vi "sync.create.vi"(8 "error in (no error)":errorcluster) -> (0 "error out":errorcluster, 3 "synchronization":refnum<class "synchronization.lvclass">)   [LabVIEW 2020, in "synchronization.lvclass"]
uses:
  synchronization.lvclass
  synchronization.lvclass/synchronization.ctl
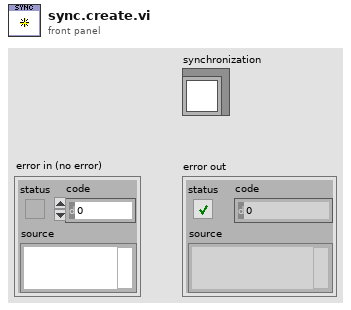
[diagram p1: front panel]
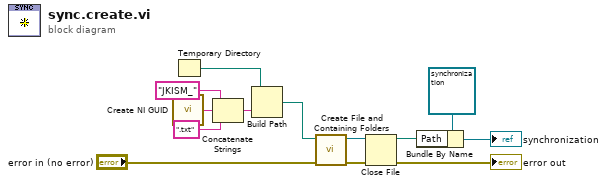
[diagram p0: block diagram]
diagram:
  n1 = call <vilib>:"Create NI GUID.vi"() -> ("NI GUID"=w11:string)
  n2 = Temporary Directory() -> (w13:path)
  n3 = Concatenate Strings("JKISM_", w11, ".txt") -> (w8:string)
  n4 = Build Path(base path=w13, name or relative path=w8) -> (appended path=w12:path)
  n5 = call <vilib>:"Create File and Containing Folders.vi"("error in (no error)"="error in (no error)", "file path"=w12) -> ("error out"=w6:errorcluster, "refnum out"=w7:refnum<file>)  [unwired: 8 in]
  n6 = Close File(refnum=w7, error in=w6) -> (path=w3:path, error out=→"error out":errorcluster)
  n7 = Bundle By Name(cluster=refnum<class "synchronization.lvclass"> refnum ("synchronization"), "Path"=w3) -> (→"synchronization":refnum<class "synchronization.lvclass">)
